vi "GPIB Find all instruments.vi"() -> (3 "Instruments":cluster{"GPIB":string, "name":string}[](array[cluster]))   [LabVIEW 2017]
uses:
  Main/Global/Flags.vi
  Main/Global/Misc.vi
panel:
  in  "endprogram":bool
  in  "clear":bool
  in  "find":bool
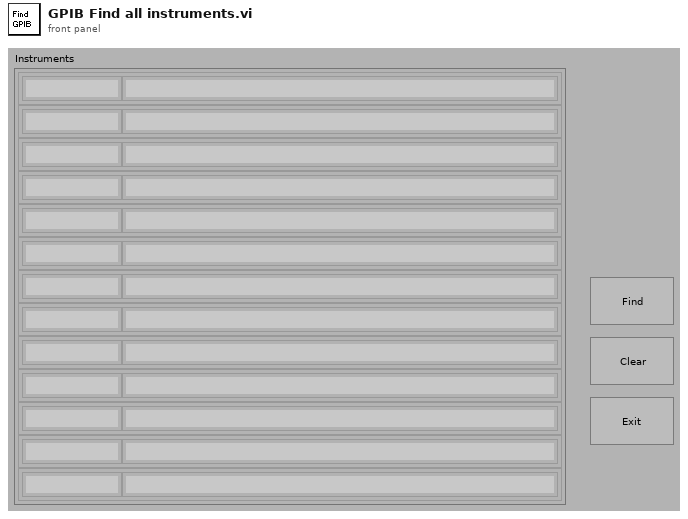
[diagram p1: front panel]
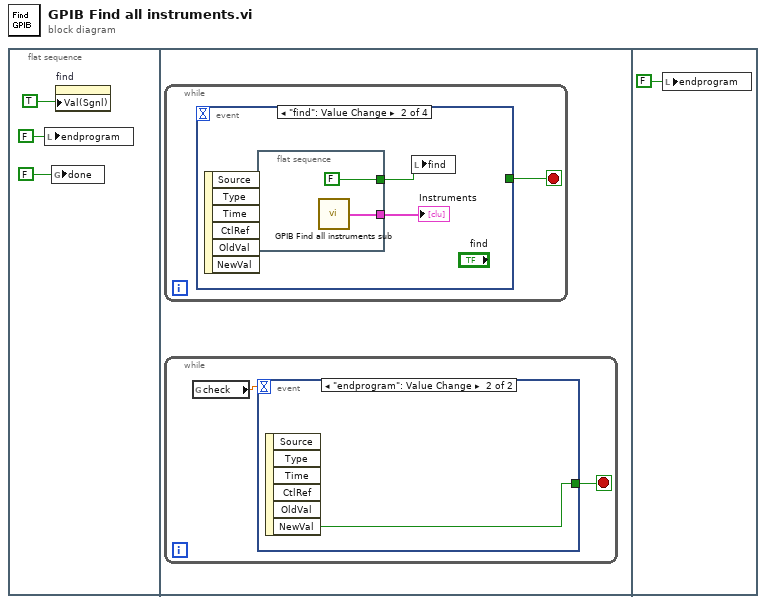
[diagram p0: block diagram]
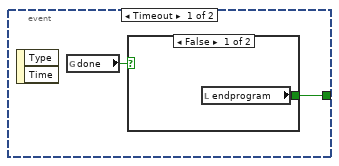
[diagram p2: hidden frame]
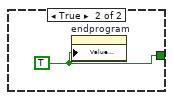
[diagram p3: hidden frame]
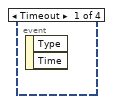
[diagram p4: hidden frame]
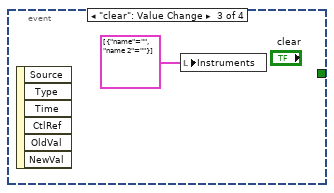
[diagram p5: hidden frame]
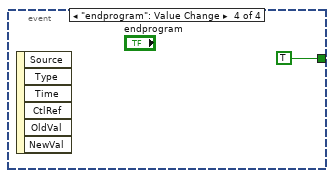
[diagram p6: hidden frame]
diagram:
  n1 = flat-sequence {
    frame #0 {
      n2 = local write "endprogram"(FALSE) -> ()
      n3 = global write "Flags.vi" "done"(FALSE) -> ()
      n4 = property on="find" class="Bool (strict)"("Val(Sgnl)"=TRUE) -> ()  [unwired: 2 in, 2 out]
    }
    frame #1 {
      n5 = while {
        stop <- w11 stop-if-true
        n6 = event shown="[1] \"find\": Value Change" {
          selector: _ -> [_ _ _ _]
          dyn-events: _ -> [_ _ _ _]
          timeout: _ -> [_ _ _ _]
          tunnel: [_ _ _ TRUE] -> w11
          event Timeout {
            n7 = event-data() -> ()  [unwired: 3 out]
          }
          event "find": Value Change {
            n8 = event-data() -> ()  [unwired: 7 out]
            n9 = flat-sequence {
              tunnel: [w15] -> w13
              tunnel: [FALSE ("find")] -> w12
              frame #0 {
                n10 = call "GPIB Find all instruments sub.vi"() -> ("Array"=w15:cluster{"GPIB Addr":string, "*IDN":string}[])
              }
            }
            n11 = local write "find"(w12) -> ()
            "Instruments" <- w13
          }
          event "clear": Value Change {
            n12 = event-data() -> ()  [unwired: 7 out]
            n13 = local write "Instruments"(cluster{"name":string, "name 2":string}[] [{"name"="", "name 2"=""}] ("instrarray")) -> ()
          }
          event "endprogram": Value Change {
            n14 = event-data() -> ()  [unwired: 7 out]
          }
        }
      }
      n15 = while {
        stop <- w5 stop-if-true
        n16 = global read "Misc.vi" "check"() -> (w4:dbl)
        n17 = event shown="[1] \"endprogram\": Value Change" {
          selector: _ -> [_ _]
          dyn-events: _ -> [_ _]
          timeout: w4 -> [_ _]
          tunnel: [w6 w10] -> w5
          event Timeout {
            n18 = event-data() -> ()  [unwired: 3 out]
            n19 = global read "Flags.vi" "done"() -> (w7:bool)
            n20 = case shown="False" w7 {
              tunnel: [w8 w9] -> w6
              frame False {
                n21 = local read "endprogram"() -> (w8:bool)
              }
              frame True {
                w9 = TRUE
                n22 = property on="endprogram" class="Bool (strict)"("Value (Signaling)"=w9) -> ()  [unwired: 2 in, 2 out]
              }
            }
          }
          event "endprogram": Value Change {
            n23 = event-data() -> ("NewVal"=w10:bool)  [unwired: 6 out]
          }
        }
      }
    }
    frame #2 {
      n24 = local write "endprogram"(FALSE) -> ()
    }
  }
